vi "Calibrate GPS Data.vi"(0 "Read Buffer":string, 2 "Latitude Error":dbl, 4 "Longitude Error":dbl, 7 "Calibrate":bool) -> (20 "Sample Time":string, 21 "Latitude":dbl format="%_13g", 22 "North or South":string, 23 "Longitude":dbl format="%_13g", 24 "East or West":string, 25 "Fixed Quality":string, 26 "Satellites Tracked":string, 27 "Altitude Above Mean Sea Level (m)":string)   [LabVIEW 2011]
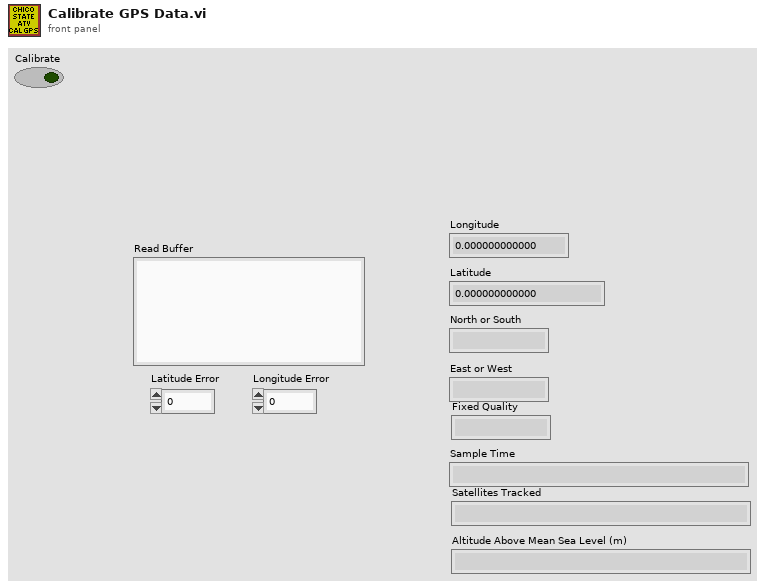
[diagram p1: front panel]
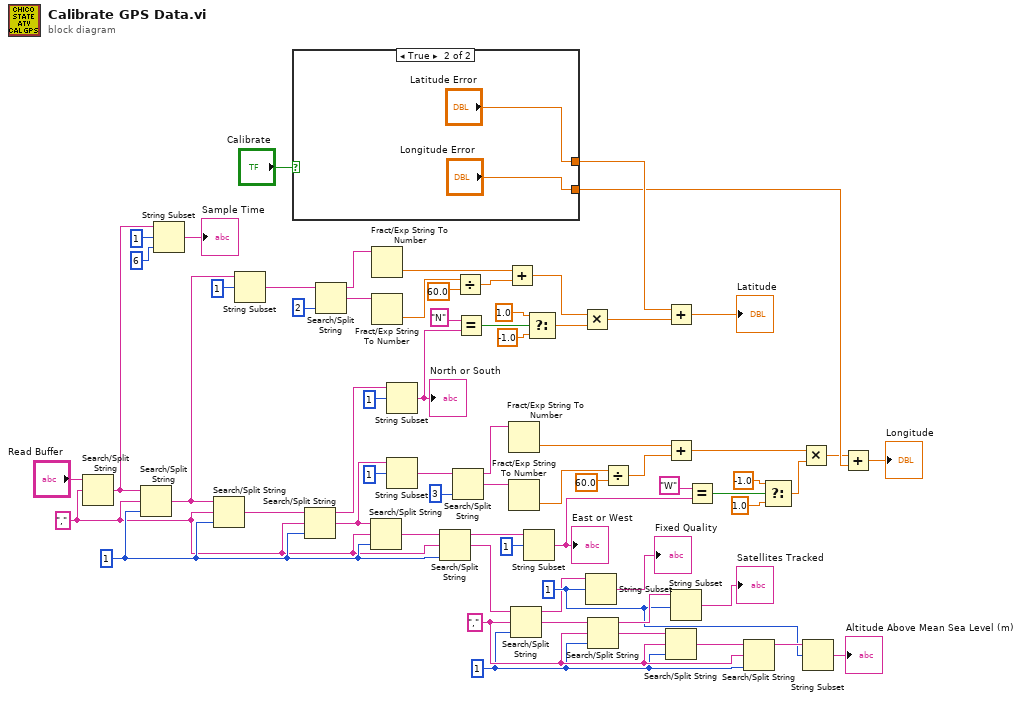
[diagram p0: block diagram]
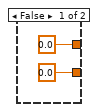
[diagram p2: hidden frame]
diagram:
  w46 = 1 ("offset (0)")
  w50 = "," ("search string/char (-)")
  w51 = 1 ("offset (0)")
  w62 = 1 ("offset (0)")
  w52 = "," ("search string/char (-)")
  n1 = Search/Split String(string="Read Buffer", search string/char (-)=w52) -> (match + rest of string=w57:string)  [unwired: 1 in, 2 out]
  n2 = Search/Split String(string=w57, search string/char (-)=w52, offset (0)=w62) -> (match + rest of string=w25:string)  [unwired: 2 out]
  n3 = String Subset(string=w57, offset (0)=1, length (rest)=6 ("length (rest)")) -> (substring=→"Sample Time":string)
  n4 = Search/Split String(string=w25, search string/char (-)=w52, offset (0)=w62) -> (match + rest of string=w63:string)  [unwired: 2 out]
  n5 = String Subset(string=w25, offset (0)=1) -> (substring=w28:string)  [unwired: 1 in]
  n6 = case shown="True" "Calibrate" {
    tunnel: [0.0 ("Latitude Error") "Latitude Error"] -> w65
    tunnel: [0.0 ("Longitude Error") "Longitude Error"] -> w64
    frame False {
    }
    frame True {
    }
  }
  n7 = Search/Split String(string=w63, search string/char (-)=w52, offset (0)=w62) -> (substring before match=w60:string, match + rest of string=w23:string)  [unwired: 1 out]
  n8 = Search/Split String(string=w28, offset (0)=2) -> (substring before match=w42:string, match + rest of string=w41:string)  [unwired: 1 in, 1 out]
  n9 = Search/Split String(string=w23, search string/char (-)=w52, offset (0)=w62) -> (match + rest of string=w24:string)  [unwired: 2 out]
  n10 = Fract/Exp String To Number(string=w42) -> (number=w38:dbl)  [unwired: 3 in, 1 out]
  n11 = Fract/Exp String To Number(string=w41) -> (number=w39:dbl)  [unwired: 3 in, 1 out]
  n12 = String Subset(string=w60, offset (0)=1 ("length (rest)")) -> (substring=w3:string)  [unwired: 1 in]
  "North or South" <- w3
  n13 = String Subset(string=w23, offset (0)=1) -> (substring=w27:string)  [unwired: 1 in]
  n14 = Search/Split String(string=w24, search string/char (-)=w52, offset (0)=w62) -> (substring before match=w61:string, match + rest of string=w47:string)  [unwired: 1 out]
  n15 = Search/Split String(string=w27, offset (0)=3) -> (substring before match=w35:string, match + rest of string=w34:string)  [unwired: 1 in, 1 out]
  n16 = Divide(x=w39, y=60.0) -> (x/y=w37:dbl)
  n17 = Equal?(x="N", y=w3) -> (x = y?=w5:bool)
  n18 = Add(x=w38, y=w37) -> (x+y=w12:dbl)
  n19 = Fract/Exp String To Number(string=w35) -> (number=w31:dbl)  [unwired: 3 in, 1 out]
  n20 = Fract/Exp String To Number(string=w34) -> (number=w32:dbl)  [unwired: 3 in, 1 out]
  n21 = Search/Split String(string=w47, search string/char (-)=w50, offset (0)=w46) -> (substring before match=w49:string, match + rest of string=w48:string)  [unwired: 1 out]
  n22 = String Subset(string=w61, offset (0)=1 ("length (rest)")) -> (substring=w17:string)  [unwired: 1 in]
  "East or West" <- w17
  n23 = Select(t=1.0, s=w5, f=-1.0) -> (s? t:f=w2:dbl)
  n24 = Multiply(x=w12, y=w2) -> (x*y=w11:dbl)
  n25 = String Subset(string=w49, offset (0)=w51) -> (substring=→"Fixed Quality":string)  [unwired: 1 in]
  n26 = Search/Split String(string=w48, search string/char (-)=w50, offset (0)=w46) -> (substring before match=w56:string, match + rest of string=w55:string)  [unwired: 1 out]
  n27 = Divide(x=w32, y=60.0) -> (x/y=w30:dbl)
  n28 = Add(x=w65, y=w11) -> (x+y=→"Latitude":dbl)
  n29 = Add(x=w31, y=w30) -> (x+y=w10:dbl)
  n30 = Search/Split String(string=w55, search string/char (-)=w50, offset (0)=w46) -> (match + rest of string=w54:string)  [unwired: 2 out]
  n31 = String Subset(string=w56, offset (0)=w51) -> (substring=→"Satellites Tracked":string)  [unwired: 1 in]
  n32 = Equal?(x="W", y=w17) -> (x = y?=w15:bool)
  n33 = Search/Split String(string=w54, search string/char (-)=w50, offset (0)=w46) -> (substring before match=w53:string)  [unwired: 2 out]
  n34 = Select(t=-1.0, s=w15, f=1.0) -> (s? t:f=w8:dbl)
  n35 = Multiply(x=w10, y=w8) -> (x*y=w9:dbl)
  n36 = String Subset(string=w53, offset (0)=w51) -> (substring=→"Altitude Above Mean Sea Level (m)":string)  [unwired: 1 in]
  n37 = Add(x=w9, y=w64) -> (x+y=→"Longitude":dbl)
